vi "Path Constants.vi"() -> (4 "Error Log Path":path, 6 "QuestionBank Drive":path, 8 "Candidates File":path)   [LabVIEW 2014, in "Coding Platform.lvlib"]
uses:
  Coding Platform.lvlib
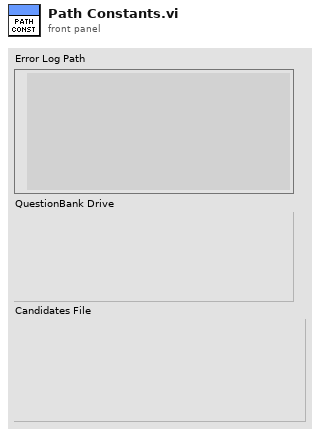
[diagram p1: front panel]
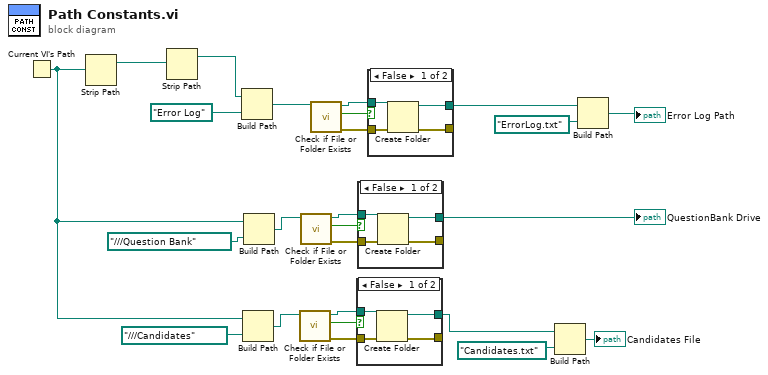
[diagram p0: block diagram]
diagram:
  n1 = Current VI's Path() -> (path=w5:path)
  n2 = Strip Path(path=w5) -> (stripped path=w25:path)  [unwired: 1 out]
  n3 = Strip Path(path=w25) -> (stripped path=w24:path)  [unwired: 1 out]
  n4 = Build Path(base path=w24, name or relative path=path "Error Log") -> (appended path=w22:path)
  n5 = Build Path(base path=w5, name or relative path=path "../../../Candidates") -> (appended path=w9:path)
  n6 = Build Path(base path=w5, name or relative path=path "../../../Question Bank") -> (appended path=w11:path)
  n7 = call <vilib>:"Check if File or Folder Exists.vi"("path"=w9) -> ("error out"=w8:errorcluster, "file or folder exists?"=w7:bool, "dup path"=w6:path)  [unwired: 8 in]
  n8 = call <vilib>:"Check if File or Folder Exists.vi"("path"=w11) -> ("error out"=w12:errorcluster, "file or folder exists?"=w13:bool, "dup path"=w14:path)  [unwired: 8 in]
  n9 = call <vilib>:"Check if File or Folder Exists.vi"("path"=w22) -> ("error out"=w21:errorcluster, "file or folder exists?"=w20:bool, "dup path"=w19:path)  [unwired: 8 in]
  n10 = case shown="False" w7 {
    tunnel: w8 -> [w29 w31]
    tunnel: w6 -> [w27 w30]
    tunnel: [w28 w31] -> _
    tunnel: [w26 w30] -> w3
    frame False {
      n11 = Create Folder(path (use dialog)=w27, error in=w29) -> (created path=w26:path, error out=w28:errorcluster)  [unwired: 1 in, 1 out]
    }
    frame True {
    }
  }
  n12 = case shown="False" w13 {
    tunnel: w12 -> [w35 w37]
    tunnel: w14 -> [w33 w36]
    tunnel: [w34 w37] -> _
    tunnel: [w32 w36] -> w10
    frame False {
      n13 = Create Folder(path (use dialog)=w33, error in=w35) -> (created path=w32:path, error out=w34:errorcluster)  [unwired: 1 in, 1 out]
    }
    frame True {
    }
  }
  "QuestionBank Drive" <- w10
  n14 = case shown="False" w20 {
    tunnel: w21 -> [w41 w43]
    tunnel: w19 -> [w39 w42]
    tunnel: [w40 w43] -> _
    tunnel: [w38 w42] -> w18
    frame False {
      n15 = Create Folder(path (use dialog)=w39, error in=w41) -> (created path=w38:path, error out=w40:errorcluster)  [unwired: 1 in, 1 out]
    }
    frame True {
    }
  }
  n16 = Build Path(base path=w3, name or relative path=path "Candidates.txt") -> (appended path=→"Candidates File":path)
  n17 = Build Path(base path=w18, name or relative path=path "ErrorLog.txt") -> (appended path=→"Error Log Path":path)
